vi "Stop Data Grid.vi"(8 "error in (no error)":errorcluster, 11 "DataGridView in":refnum<class "DataGridView.lvclass">) -> (0 "error out":errorcluster, 3 "DataGridView out":refnum<class "DataGridView.lvclass">)   [LabVIEW 2013, in "DataGrid.lvlib" / "DataGridView.lvclass"]
doc: "This VI must be called to properly stop the grid, as it unregisters the .net callback events, that otherwise, stay running and lock the classes."
uses:
  DataGridView.lvclass
  System.Windows.Forms
  System.Data
  DataTable/DataTable.lvclass
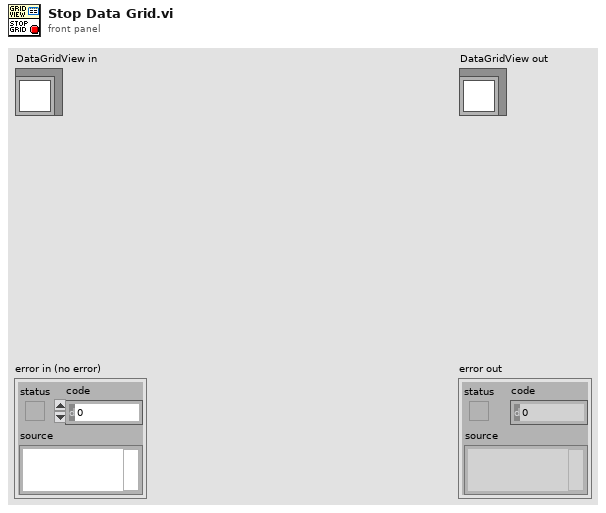
[diagram p1: front panel]
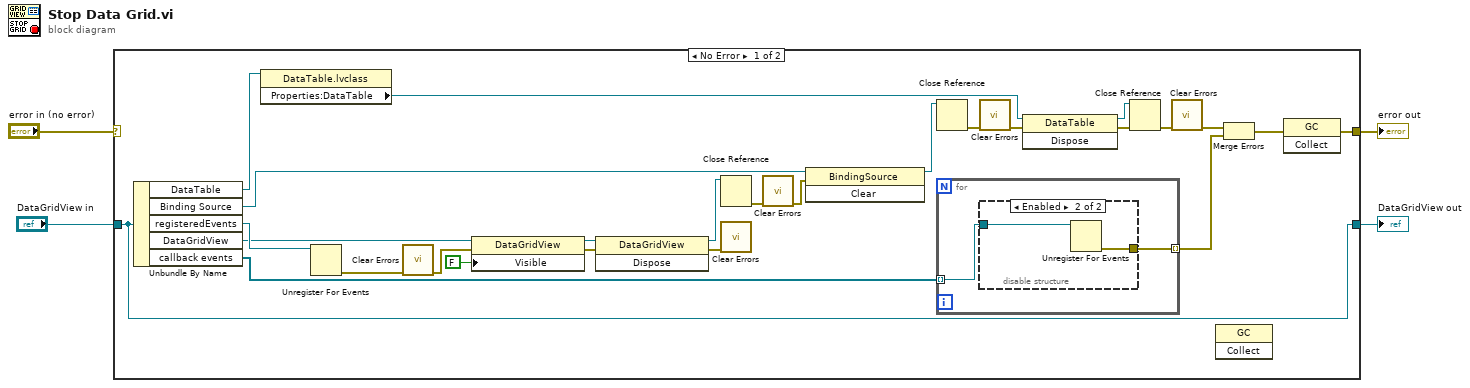
[diagram p0: block diagram]
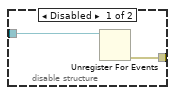
[diagram p2: hidden frame]
diagram:
  n1 = case shown="No Error" "error in (no error)" {
    selector: "error in (no error)" -> [_ w38]
    tunnel: [w26 w38] -> w3
    tunnel: [w30 w37] -> w1
    tunnel: "DataGridView in" -> [w30 w37]
    frame No Error {
      n2 = Unbundle By Name(w30) -> ("DataTable"=w25:refnum<class "DataTable.lvclass">, "Binding Source"=w22:refnum<k24>, "registeredEvents"=w24:refnum<event-registration>, "DataGridView"=w23:refnum<k24>, "callback events"=w29:refnum<k27>[])
      n3 = property class="DataTable.lvclass"(reference=w25) -> ("Properties:DataTable"=w21:refnum<k24>)  [unwired: 1 in, 2 out]
      n4 = Unregister For Events(event registration refnum=w24) -> (error out=w18:errorcluster)  [unwired: 1 in]
      n5 = call <vilib>:"Clear Errors.vi"("error in (no error)"=w18) -> ("error out"=w6:errorcluster)  [unwired: 5 in, 1 out]
      n6 = property class="DataGridView"(reference=w23, error in=w6, "Visible"=FALSE) -> (reference out=w15:refnum<k24>, error out=w14:errorcluster)
      n7 = invoke class="DataGridView" method="Dispose"(reference=w15, error in=w14) -> (reference out=w17:refnum<k24>, error out=w12:errorcluster)  [unwired: 1 in, 1 out]
      n8 = Close Reference(reference=w17) -> (error out=w13:errorcluster)  [unwired: 1 in]
      n9 = call <vilib>:"Clear Errors.vi"("error in (no error)"=w12) -> ()  [unwired: 5 in, 2 out]
      n10 = call <vilib>:"Clear Errors.vi"("error in (no error)"=w13) -> ("error out"=w20:errorcluster)  [unwired: 5 in, 1 out]
      n11 = invoke class="BindingSource" method="Clear"(reference=w22, error in=w20) -> (reference out=w11:refnum<k24>)  [unwired: 1 in, 2 out]
      n12 = Close Reference(reference=w11) -> (error out=w10:errorcluster)  [unwired: 1 in]
      n13 = for {
        tunnel: w29 -> [w32] mode=indexing
        tunnel: [w31] -> w28 mode=indexing
        n14 = disable-structure shown="Enabled" {
          disable-tunnel: w32 -> [w34 w36]
          disable-tunnel: [w33 w35] -> w31
          frame Disabled {
            n15 = Unregister For Events(event registration refnum=w34) -> (error out=w33:errorcluster)  [unwired: 1 in]
          }
          frame Enabled {
            n16 = Unregister For Events(event registration refnum=w36) -> (error out=w35:errorcluster)  [unwired: 1 in]
          }
        }
      }
      n17 = call <vilib>:"Clear Errors.vi"("error in (no error)"=w10) -> ("error out"=w19:errorcluster)  [unwired: 5 in, 1 out]
      n18 = invoke class="DataTable" method="Dispose"(reference=w21, error in=w19) -> (reference out=w7:refnum<k24>, error out=w9:errorcluster)  [unwired: 1 in, 1 out]
      n19 = Close Reference(reference=w7, error in (no error)=w9) -> (error out=w8:errorcluster)
      n20 = call <vilib>:"Clear Errors.vi"("error in (no error)"=w8) -> ("error out"=w5:errorcluster)  [unwired: 5 in, 1 out]
      n21 = invoke class="GC" method="Collect"() -> ()  [unwired: 3 in, 3 out]
      n22 = Merge Errors(w5, w28) -> (w27:errorcluster)
      n23 = invoke class="GC" method="Collect"(error in=w27) -> (error out=w26:errorcluster)  [unwired: 2 in, 2 out]
    }
    frame Error {
    }
  }
  "error out" <- w3
  "DataGridView out" <- w1
